vi "Actor Core.vi"(8 "error in":errorcluster, 11 "Nested in":refnum<class "Counter.lvclass">) -> (0 "error out":errorcluster, 3 "Actor out":refnum<class "Actor.lvclass">)   [LabVIEW 2019, in "Counter.lvlib" / "Counter.lvclass"]
doc: "(<B>Filename</B>: Actor Framework.lvlib:Actor.lvclass:Actor Core.vi)\n\nReceives messages to the actor, reacts to them, and initiates any error handling that may shut the actor down.\n\nDescendant classes may override this VI to append parallel tasks for the actor to complete while it handles messages. Overrides use the Call Parent Method node."
uses:
  Counter.lvclass
  C:/Program Files/National Instruments/LabVIEW 2019/vi.lib/ActorFramework/Actor/Actor.lvclass
  <vilib>/ActorFramework/Actor/Actor.lvclass
  Counter ACQ/Counter ACQ.lvclass
  Counter.lvclass/Counter.ctl
  <vilib>/ActorFramework/Actor/Actor.lvclass/Actor.ctl
  <vilib>/ActorFramework/Message Enqueuer/Message Enqueuer.lvclass/Message Enqueuer.ctl
  Counter Messages/StartStop Msg/StartStop Msg.lvclass/StartStop Msg.ctl
  Counter Messages/Maximo Msg/Maximo Msg.lvclass/Maximo Msg.ctl
  Counter Messages/Minimo Msg/Minimo Msg.lvclass/Minimo Msg.ctl
  <vilib>/ActorFramework/Message Enqueuer/Init from Existing Queue.vi
  <vilib>/ActorFramework/Message Enqueuer/Enqueue.vi
  <vilib>/Utility/error.llb/Clear Errors.vi
  <vilib>/ActorFramework/Stop Msg/Stop Msg.lvclass
  C:/Program Files/National Instruments/LabVIEW 2019/vi.lib/ActorFramework/Message/Message.lvclass
  Counter Messages/StartStop Msg/StartStop Msg.lvclass
  Counter Messages/Maximo Msg/Maximo Msg.lvclass
  Counter Messages/Minimo Msg/Minimo Msg.lvclass
  <vilib>/ActorFramework/Message Priority Queue/Priority Enqueue.vi
  <vilib>/ActorFramework/Message Enqueuer/Message Enqueuer.lvclass
panel:
  out "Leds":bool[](array[boolean])
  in  "Maximo":dbl
  in  "Minimo":dbl
  in  "Save":bool
  in  "Format":enum16{"select", "txt", "tdms"}(ring)
  in  "Path":path
  in  "Stop":bool
  in  "Start":bool
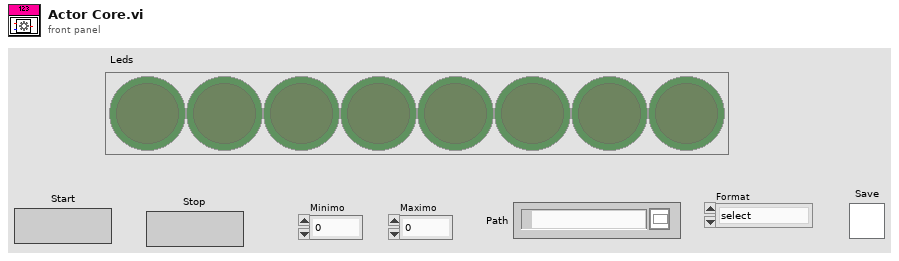
[diagram p1: front panel]
types:
  T1 = cluster{"Stop":refnum<user-event>, "Leds":refnum<user-event>}
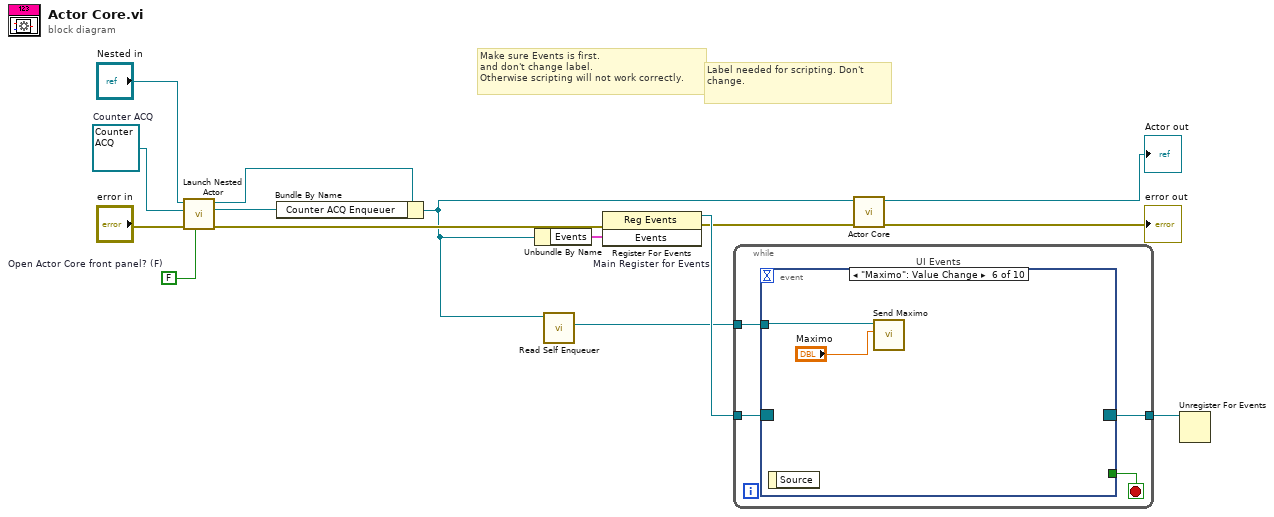
[diagram p0: block diagram]
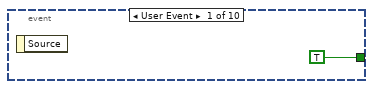
[diagram p2: hidden frame]
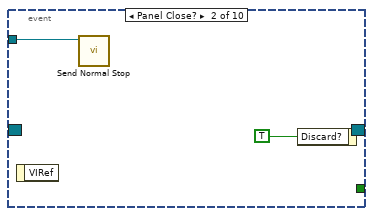
[diagram p3: hidden frame]
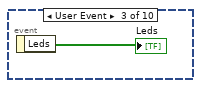
[diagram p4: hidden frame]
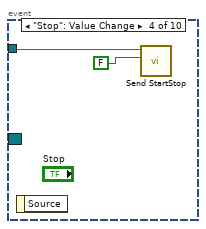
[diagram p5: hidden frame]
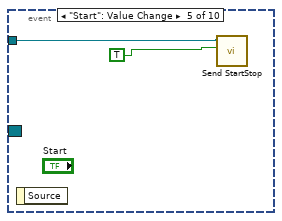
[diagram p6: hidden frame]
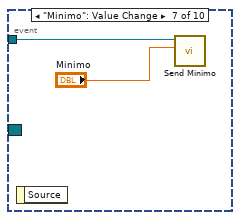
[diagram p7: hidden frame]
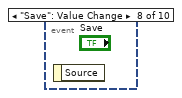
[diagram p8: hidden frame]
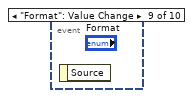
[diagram p9: hidden frame]
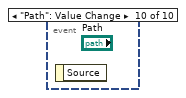
[diagram p10: hidden frame]
diagram:
  w1 = FALSE  # Open Actor Core front panel? (F)
  w5 = refnum<class "Counter ACQ.lvclass"> refnum  # Counter ACQ
  # "Label needed for scripting. Don't change."
  # "Make sure Events is first.\nand don't change label.\nOtherwise scripting will not work correctly."
  n1 = call <vilib>:"Launch Nested Actor.vi"("Open Actor Core front panel? (F)"=w1, "error in (no error)"="error in", "Nested Actor"=w5, "Caller Actor in"="Nested in") -> ("error out"=w7:errorcluster, "Nested Actor's Enqueuer"=w4:refnum<class "Message Enqueuer.lvclass">, "Caller Actor out"=w3:refnum<class "Counter.lvclass">)  [unwired: 5 in]
  n2 = Bundle By Name(cluster=w3, "Counter ACQ Enqueuer"=w4) -> (w2:refnum<class "Counter.lvclass">)
  n3 = Unbundle By Name(w2) -> ("Events"=w12:T1)
  n4 = call <vilib>:"Read Self Enqueuer.vi"("Actor"=w2) -> ("Self Enqueuer"=w10:refnum<class "Message Enqueuer.lvclass">)  [unwired: 10 in]
  n5 = register-events "Main Register for Events"(error in=w7, w12) -> (reference out=w13:refnum<event-registration>, error out=w9:errorcluster)  [unwired: 1 in]
  n6 = while {
    tunnel: w13 -> [w19]
    tunnel: [w17] -> w11
    tunnel: w10 -> [w16]
    stop <- w18 stop-if-true
    n7 = event "UI Events" shown="[5] \"Maximo\": Value Change" {
      selector: w19 -> [_ _ _ _ _ _ _ _ _ _]
      dyn-events: [_ _ _ _ _ _ _ _ _ _] -> w17
      timeout: _ -> [_ _ _ _ _ _ _ _ _ _]
      tunnel: [TRUE _ _ _ _ _ _ _ _ _] -> w18
      tunnel: w16 -> [_ w21 _ w25 w27 w29 w31 _ _ _]
      event User Event {
        n8 = event-data() -> ()  [unwired: 1 in, 1 out]
      }
      event Panel Close? {
        n9 = event-data() -> ()  [unwired: 1 in, 1 out]
        n10 = call <vilib>:"Send Normal Stop.vi"("Message Enqueuer"=w21) -> ()  [unwired: 10 in, 1 out]
        n11 = event-data("Discard?"=TRUE) -> ()  [unwired: 1 in, 1 out]
      }
      event User Event {
        n12 = event-data() -> ("Leds"=→"Leds":bool[])  [unwired: 1 in]
      }
      event "Stop": Value Change {
        n13 = event-data() -> ()  [unwired: 1 in, 1 out]
        n14 = call "Send StartStop.vi"("Start/Stop"=FALSE ("Stop"), "Message Enqueuer"=w25) -> ()  [unwired: 8 in, 2 out]
      }
      event "Start": Value Change {
        n15 = event-data() -> ()  [unwired: 1 in, 1 out]
        n16 = call "Send StartStop.vi"("Start/Stop"=TRUE ("Start"), "Message Enqueuer"=w27) -> ()  [unwired: 8 in, 2 out]
      }
      event "Maximo": Value Change {
        n17 = event-data() -> ()  [unwired: 1 in, 1 out]
        n18 = call "Send Maximo.vi"("Maximo"="Maximo", "Message Enqueuer"=w29) -> ()  [unwired: 8 in, 2 out]
      }
      event "Minimo": Value Change {
        n19 = event-data() -> ()  [unwired: 1 in, 1 out]
        n20 = call "Send Minimo.vi"("Minimo"="Minimo", "Message Enqueuer"=w31) -> ()  [unwired: 8 in, 2 out]
      }
      event "Save": Value Change {
        n21 = event-data() -> ()  [unwired: 1 in, 1 out]
      }
      event "Format": Value Change {
        n22 = event-data() -> ()  [unwired: 1 in, 1 out]
      }
      event "Path": Value Change {
        n23 = event-data() -> ()  [unwired: 1 in, 1 out]
      }
    }
  }
  n24 = call-parent "Actor Core.vi"("error in"=w9, "Actor in"=w2) -> ("error out"=→"error out":errorcluster, "Actor out"=→"Actor out":refnum<class "Actor.lvclass">)  [unwired: 8 in]
  n25 = Unregister For Events(event registration refnum=w11) -> ()  [unwired: 1 in, 1 out]
